vi "PH_GUI.set I32 ring GUI object.vi"(2 "Ring Ref":refnum<vi>, 3 "Value":i32, 4 "Blinking (false)":bool, 5 "error in (no error)":errorcluster) -> (19 "error out":errorcluster)   [LabVIEW 2014, in "PH_Common.lvlib"]
doc: "Sets value and more for the referenced GUI object."
uses:
  PH_Common.lvlib
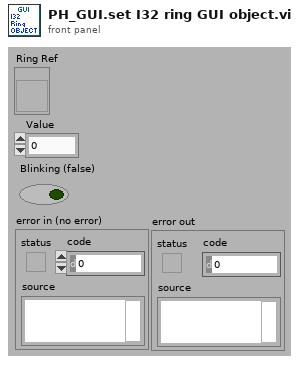
[diagram p1: front panel]
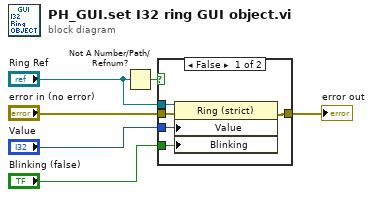
[diagram p0: block diagram]
diagram:
  n1 = Not A Number/Path/Refnum?(number/path/refnum="Ring Ref") -> (NaN/Path/Refnum?=w5:bool)
  n2 = case shown="False" w5 {
    tunnel: "error in (no error)" -> [w10 w12]
    tunnel: "Ring Ref" -> [w11 _]
    tunnel: "Value" -> [w7 _]
    tunnel: "Blinking (false)" -> [w8 _]
    tunnel: [w9 w12] -> w2
    frame False {
      n3 = property class="Ring (strict)"(reference=w11, error in=w10, "Value"=w7, "Blinking"=w8) -> (error out=w9:errorcluster)  [unwired: 1 out]
    }
    frame True {
    }
  }
  "error out" <- w2
